vi "svm_set_print_function.vi"(8 "error in (no error)":errorcluster, 11 "Logging event":refnum<user-event>) -> (0 "error out":errorcluster, 3 "Logging event duplicate":refnum<user-event>)   [LabVIEW 2014]
uses:
  bin/x64/LVLibSVM.dll
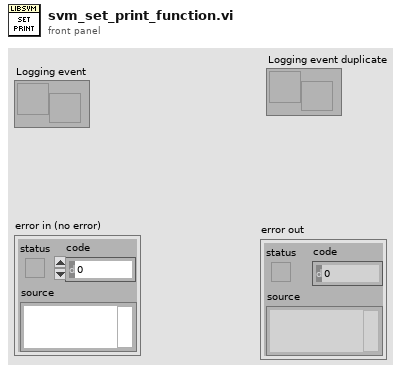
[diagram p1: front panel]
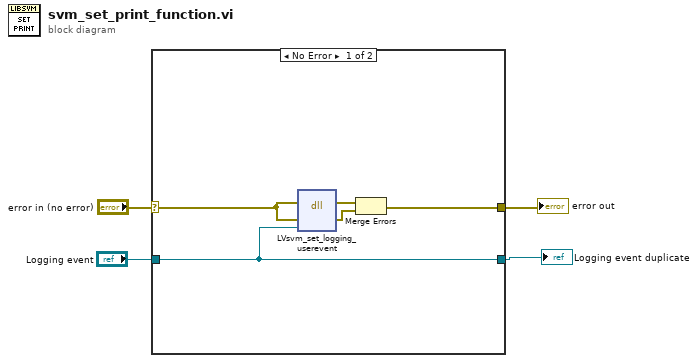
[diagram p0: block diagram]
diagram:
  n1 = case shown="No Error" "error in (no error)" {
    selector: "error in (no error)" -> [w6 w11]
    tunnel: [w7 w11] -> w4
    tunnel: "Logging event" -> [w5 w10]
    tunnel: [w5 w10] -> w2
    frame No Error {
      n2 = dll-call lib="C:/dev/LabVIEW-libsvm/LabVIEW/bin/x64/LVLibSVM.dll" fn="LVsvm_set_logging_userevent"(error in=w6, "lvErr"=w6, "loggingUsrEvent"=w5) -> (error out=w9:errorcluster, "lvErr"=w8:errorcluster)  [unwired: 4 in, 1 out]
      n3 = Merge Errors(w9, w8) -> (w7:errorcluster)
    }
    frame Error {
    }
  }
  "error out" <- w4
  "Logging event duplicate" <- w2
